vi "Erase State History.vi"(8 "State Control History In":T1[](array[typedef]), 10 "Erase History? (f)":bool, 11 "State Control Times In":string[](array[string])) -> (0 "State Control History Out":T1[](array[typedef]), 3 "State Control Times Out":string[](array[string]))   [LabVIEW 2016]
uses:
  Types/State Control.ctl
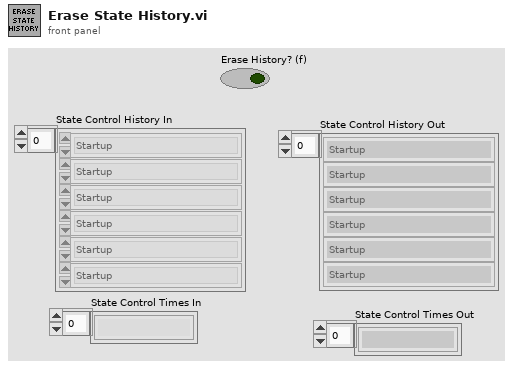
[diagram p1: front panel]
types:
  T1 = typedef "State Control.ctl" = enum16{"Startup", "Read Config File", "Initilize Optional Hardware", "Idle", "New Session", "Read GUI Pars", "Configure Hardware", "Initialize Set", "Pre-Scan", "Scan", "Post-Scan", "Exit Set", "Automated Tuning", "Manual Tuning", "Check Calibration", "Optimize RF Power", "Test Scan", "Set Oxy QA-Scan Pars", "Find Peaks", "Update from Cursors", "Flag Bad Set", "Mark transition time", "Measure Q", "Measure Noise", "Rotate Magnet", "Lock Field", "Engineering Tuning", "Zero Voltages", "Update Center Field", "Refit Data", "Open Session Data Folder", "AfterSave", "Undo Auto Update Pars", "Read from Script", "End Session", "Quit Software", "Error"}
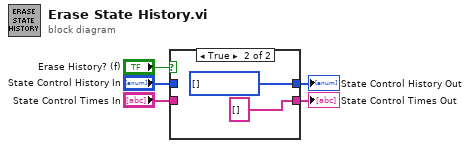
[diagram p0: block diagram]
diagram:
  n1 = case shown="True" "Erase History? (f)" {
    tunnel: [w7 w9] -> w5
    tunnel: [w6 string[] [] ("State Control Times Out")] -> w4
    tunnel: "State Control History In" -> [w7 _]
    tunnel: "State Control Times In" -> [w6 _]
    frame False {
    }
    frame True {
      w9 = T1[] [] items=["Startup", "Read Config File", "Initilize Optional Hardware", "Idle", "New Session", "Read GUI Pars", "Configure Hardware", "Initialize Set", "Pre-Scan", "Scan", "Post-Scan", "Exit Set", "Automated Tuning", "Manual Tuning", "Check Calibration", "Optimize RF Power", "Test Scan", "Set Oxy QA-Scan Pars", "Find Peaks", "Update from Cursors", "Flag Bad Set", "Mark transition time", "Measure Q", "Measure Noise", "Rotate Magnet", "Lock Field", "Engineering Tuning", "Zero Voltages", "Update Center Field", "Refit Data", "Open Session Data Folder", "AfterSave", "Undo Auto Update Pars", "Read from Script", "End Session", "Quit Software", "Error"] ("State Control History Out")
    }
  }
  "State Control History Out" <- w5
  "State Control Times Out" <- w4
